vi "sub_cam-main.vi"(8 "error in":errorcluster) -> (0 "error out":errorcluster)   [LabVIEW 2016]
uses:
  Global.vi
  <vilib>/Analysis/NI_AALPro.lvlib
panel:
  out "Image Pixels (I16)":i16[][](array[numeric])
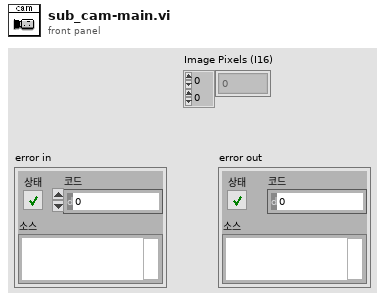
[diagram p1: front panel]
types:
  T1 = cluster{"Global Rectangle":i32[], "Contours":cluster{"Contour Type":u32, "ROI Type":u32, "Points":i32[]}[]}
  T2 = typedef "IMAQ Image.ctl" = refnum<image>
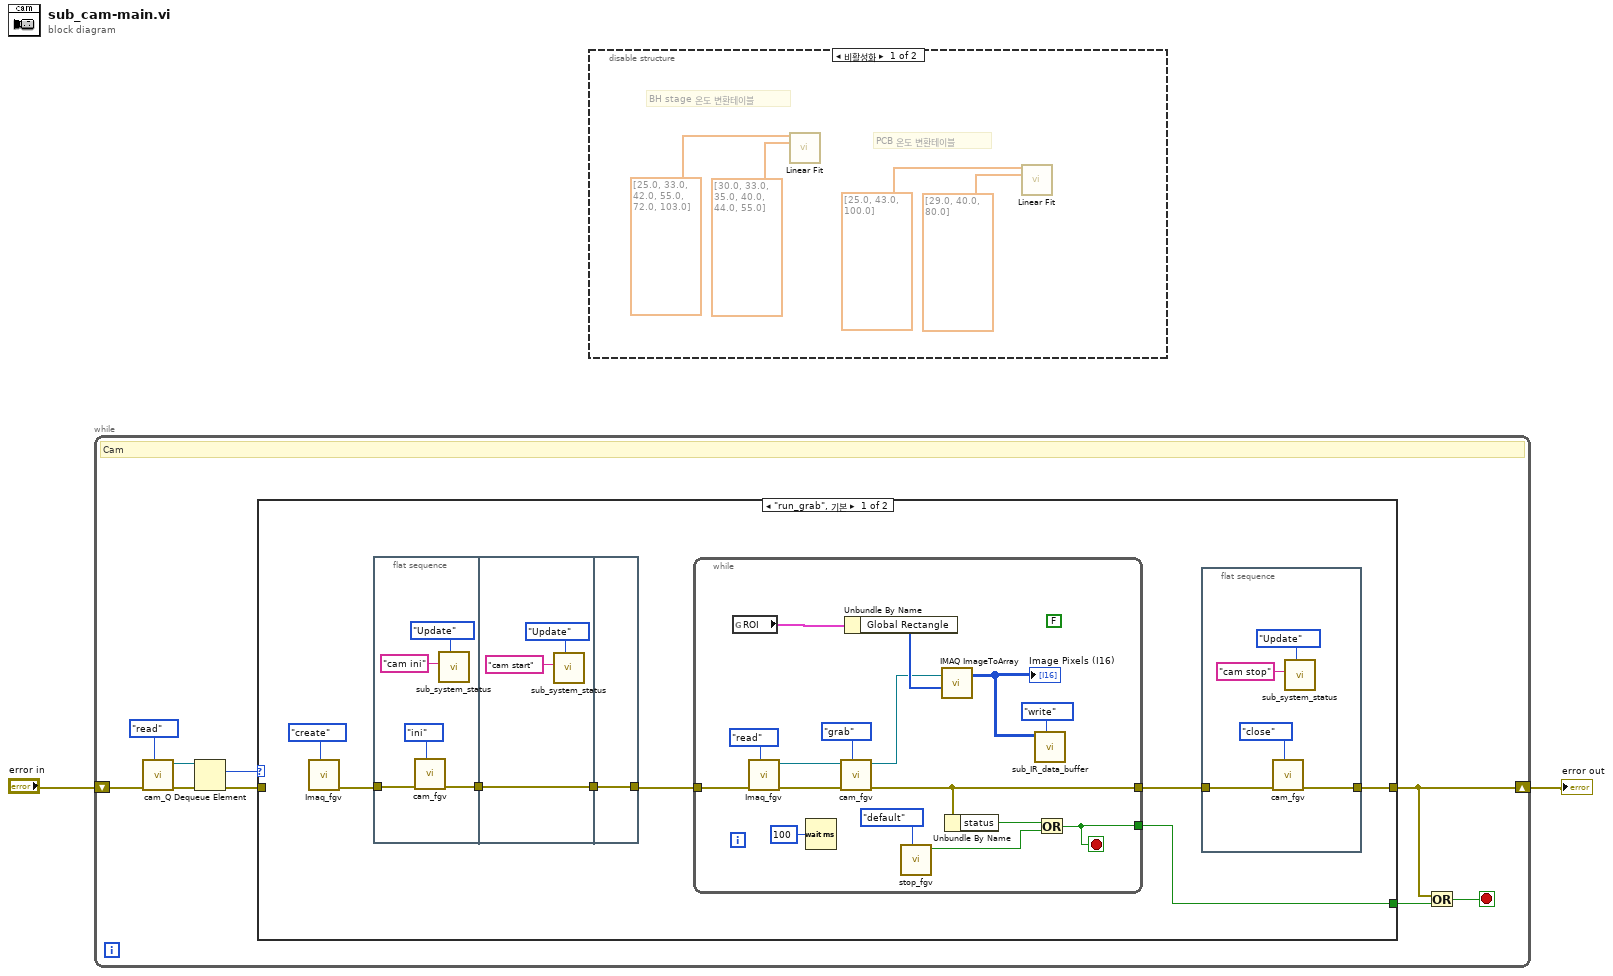
[diagram p0: block diagram]
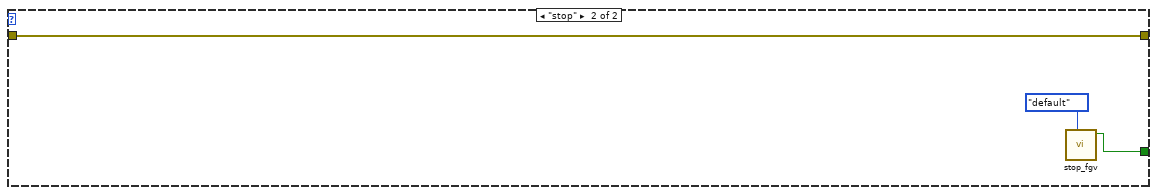
[diagram p3: hidden frame]
diagram:
  n1 = while {
    shift-right: [w3] -> w1
    shift-left: "error in" -> [w6]
    stop <- w4 stop-if-true
    # "Cam"
    n2 = call "cam_Q.vi"("cmd"=enum16{"create", "write", "read", "close"}."read", "error in"=w6) -> ("error out"=w10:errorcluster, "queue out"=w9:refnum<queue>)  [unwired: 8 in]
    n3 = Dequeue Element(queue=w9, error in (no error)=w10) -> (element=w7:enum16{"run_grab", "stop"}, error out=w8:errorcluster)  [unwired: 1 in, 2 out]
    n4 = case shown="\"run_grab\", 기본" w7 {
      tunnel: w8 -> [_ w52]
      tunnel: [w14 w50] -> w5
      tunnel: [w15 w52] -> w3
      frame "run_grab", Default {
        n5 = call "Imaq_fgv.vi"("cmd"=enum16{"create", "close", "read"}."create") -> ("error out"=w19:errorcluster)  [unwired: 9 in, 1 out]
        n6 = flat-sequence {
          tunnel: w19 -> [w29]
          tunnel: [w27] -> w13
          tunnel: w13 -> [w32]
          tunnel: [w32] -> w12
          tunnel: [w33] -> w17
          tunnel: w12 -> [w33]
          frame #0 {
            n7 = call "cam_fgv.vi"("cmd"=enum16{"ini", "grab", "close"}."ini", "error in"=w29) -> ("error out"=w27:errorcluster)  [unwired: 8 in, 1 out]
            n8 = call "sub_system_status.vi"("Mode"=enum16{"Initial", "Update", "Clear"}."Update", "String in"="cam ini") -> ()  [unwired: 9 in, 1 out]
          }
          frame #1 {
            n9 = call "sub_system_status.vi"("Mode"=enum16{"Initial", "Update", "Clear"}."Update", "String in"="cam start") -> ()  [unwired: 9 in, 1 out]
          }
          frame #2 {
          }
        }
        n10 = while {
          tunnel: w17 -> [w39]
          tunnel: [w45] -> w16
          tunnel: [w47] -> w14
          stop <- w47 stop-if-true
          (unwired) FALSE
          n11 = global read "Global.vi" "ROI"() -> (w41:T1)
          n12 = call "Imaq_fgv.vi"("cmd"=enum16{"create", "close", "read"}."read", "error in"=w39) -> ("error out"=w38:errorcluster, "New Image"=w37:T2)  [unwired: 8 in]
          n13 = Wait (ms)(milliseconds to wait=u32 100 ("대기 시간(ms)")) -> ()  [unwired: 1 out]
          n14 = call "cam_fgv.vi"("cmd"=enum16{"ini", "grab", "close"}."grab", "error in"=w38, "Image In"=w37) -> ("error out"=w45:errorcluster, "Image Out"=w36:T2)  [unwired: 7 in]
          n15 = Unbundle By Name(w41) -> ("Global Rectangle"=w48:i32[])
          n16 = call "stop_fgv.vi"("cmd"=enum16{"default", "ini", "stop"}."default") -> ("stop"=w42:bool)  [unwired: 9 in, 1 out]
          n17 = call "IMAQ ImageToArray"("Optional Rectangle"=w48, "Image"=w36) -> ("Image Pixels (I16)"=w35:i16[][])  [unwired: 2 in, 4 out]
          "Image Pixels (I16)" <- w35
          n18 = Unbundle By Name(w45) -> ("status"=w49:bool)
          n19 = call "sub_IR_data_buffer.vi"("cmd"=enum16{"write", "read"}."write", "IR data"=w35) -> ()  [unwired: 9 in, 1 out]
          n20 = Or(x=w49, y=w42) -> (x .or. y?=w47:bool)
        }
        n21 = flat-sequence {
          tunnel: w16 -> [w23]
          tunnel: [w22] -> w15
          frame #0 {
            n22 = call "cam_fgv.vi"("cmd"=enum16{"ini", "grab", "close"}."close", "error in"=w23) -> ("error out"=w22:errorcluster)  [unwired: 8 in, 1 out]
            n23 = call "sub_system_status.vi"("Mode"=enum16{"Initial", "Update", "Clear"}."Update", "String in"="cam stop") -> ()  [unwired: 9 in, 1 out]
          }
        }
      }
      frame "stop" {
        n24 = call "stop_fgv.vi"("cmd"=enum16{"default", "ini", "stop"}."default") -> ("stop"=w50:bool)  [unwired: 9 in, 1 out]
      }
    }
    n25 = Or(x=w3, y=w5) -> (x .or. y?=w4:bool)
  }
  "error out" <- w1
  n26 = disable-structure shown="비활성화" {
    frame Disabled {
      # "PCB 온도 변환테이블"
      # "BH stage 온도 변환테이블"
      n27 = call <vilib>:"Linear Fit.vi"("Y"=dbl[] [25.0, 33.0, 42.0, 55.0, 72.0, 103.0] ("X"), "X"=dbl[] [30.0, 33.0, 35.0, 40.0, 44.0, 55.0]) -> ()  [unwired: 9 in, 5 out]
      n28 = call <vilib>:"Linear Fit.vi"("Y"=dbl[] [25.0, 43.0, 100.0] ("X"), "X"=dbl[] [29.0, 40.0, 80.0]) -> ()  [unwired: 9 in, 5 out]
    }
    frame Enabled {
    }
  }
